vi "Angle Offset Calculator.vi"(4 "Basket forward offset":dbl, 6 "Camera forward of turret":dbl, 8 "error in (no error)":errorcluster, 9 "Target Distance":dbl, 10 "Basket X offset":dbl, 11 "Turret Gyro (Radians)":dbl) -> (0 "error out":errorcluster, 2 "Distance":dbl, 3 "Angle Offset":dbl)   [LabVIEW 2011]
uses:
  <vilib>/Analysis/coordinate.llb/2D Cartesian Coordinate Rotation (Scalar).vi
  <vilib>/Analysis/NI_AALPro.lvlib
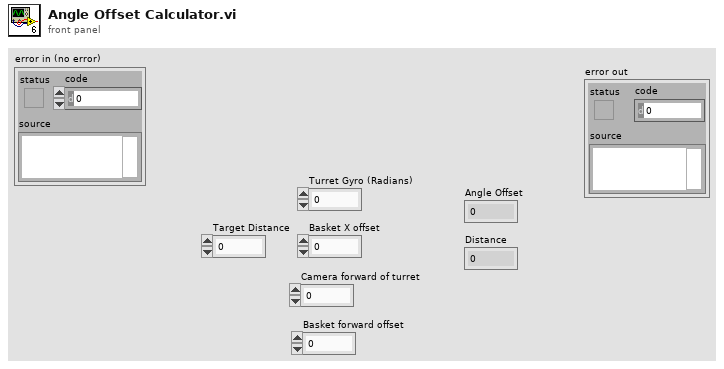
[diagram p1: front panel]
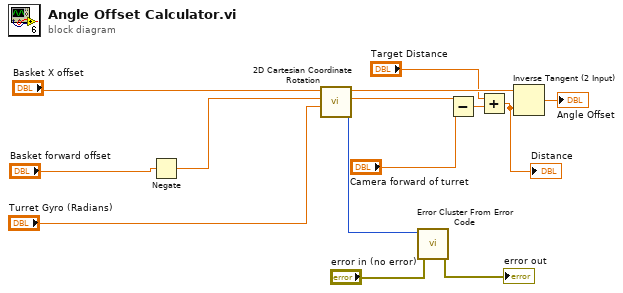
[diagram p0: block diagram]
diagram:
  n1 = Negate(x="Basket forward offset") -> (-x=w4:dbl)
  n2 = call-poly <vilib>:"2D Cartesian Coordinate Rotation.vi"("theta"="Turret Gyro (Radians)", "y"=w4, "x"="Basket X offset") -> ("error"=w13:i32, "y out"=w8:dbl, "x out"=w7:dbl)  [unwired: 6 in]
  n3 = call <vilib>:"Error Cluster From Error Code.vi"("error in (no error)"="error in (no error)", "error code (0)"=w13) -> ("error out"=→"error out":errorcluster)  [unwired: 7 in]
  n4 = Subtract(x=w8, y="Camera forward of turret") -> (x-y=w3:dbl)
  n5 = Add(x="Target Distance", y=w3) -> (x+y=w2:dbl)
  "Distance" <- w2
  n6 = Inverse Tangent (2 Input)(1:w2, 2:w7) -> (0:→"Angle Offset":dbl)
